vi "PASSCMNdll.vi"(8 "error in (no error)":errorcluster, 11 "Inputs":T2) -> (0 "error out":errorcluster, 3 "Outputs":T1)   [LabVIEW 2016]
doc: "subroutine PASSCMN(hvr, iset, icomp, jcomp, hstr, ilng, dbl, arr, ierr, herr, hvr_length, hstr_length,\nherr_length)\n\nGet or set values of variables in the common blocks.\n\nExamples:\nCall PASSCMN ('txeos', 0,3,0, h,i, tmx,z, ierr,herr) - get tmax of component 3\nCall PASSCMN ('deos', 1,2,0, h,i, dmx,z, ierr,herr) - set dmax of component 2\nCall PASSCMN ('tz', 0,1,0, h,i, tc, z, ierr,herr) - get reducing temperature of component 1\nCall PASSCMN ('ntermf', 0,1,0, h,nt,v, z, ierr,herr) - get number of terms in the Helmholtz equation for component 1\nCall PASSCMN ('coefhmx',1,1,0, h,i, v, cf, ierr,herr) - set the coefficients in the Helmholtz equation for component 1\nCall PASSCMN ('cpc0', 1,5,0, h,i, v, cp0, ierr,herr) - set the coefficients in the cp0 equation for component 5\nCall PASSCMN ('fprkij', 1,1,2, h,i, v, fpr, ierr,herr) - set the PR coefficient for the 1,2 binary\n\nINPUTS:\nhvr --character string with the common variable's name (lower case only)\niset --flag to indicate the get/set condition\n 0 - get variable value\n 1 - set variable value\nicomp --component number\njcomp --second component number for binary mixture variables\nhstr --input for a character string\nilng --input for a long variable\ndbl --input for a double precision variable\narr --input for a double precision array\n note: values in this array are not initialized to 0\n\nOUTPUTS:\nhstr -- output for a character string\nilng -- output for a long variable\ndbl -- output for a double precision variable\narr -- output for a double precision array\n note: values in this array are not initialized to 0\nierr -- error flag: \n 0 = successful\n 1 = unrecognized variable name\nherr -- error string (character*255 variable if ierr<>0)\nhvr_length -- length of variable hvr (default: -1)\nhstr_length -- length of variable hstr (default: 255)\nherr_length -- length of variable herr (default: 255)"
uses:
  REFPROP.DLL
panel:
  # "REFPROP-PASSCMNdll.vi"
  # "void  PASSCMN(CStr hvr, int32_t *iset, int32_t *icomp, int32_t *jcomp, CStr hstr, int32_t *iling, double *dbl, double *arr, int32_t *ierr, CStr herr, int32_t hvr_length, int32_t hstr_length, int32_t herr_length)"
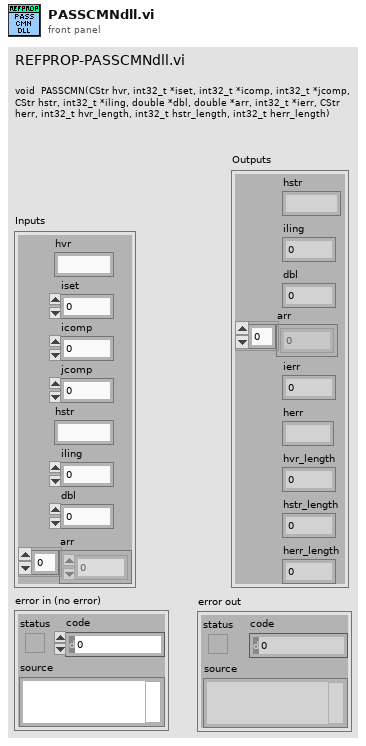
[diagram p1: front panel]
types:
  T1 = cluster{"hstr":string, "iling":i32, "dbl":dbl, "arr":dbl[], "ierr":i32, "herr":string, "hvr_length":i32, "hstr_length":i32, "herr_length":i32}
  T2 = cluster{"hvr":string, "iset":i32, "icomp":i32, "jcomp":i32, "hstr":string, "iling":i32, "dbl":dbl, "arr":dbl[]}
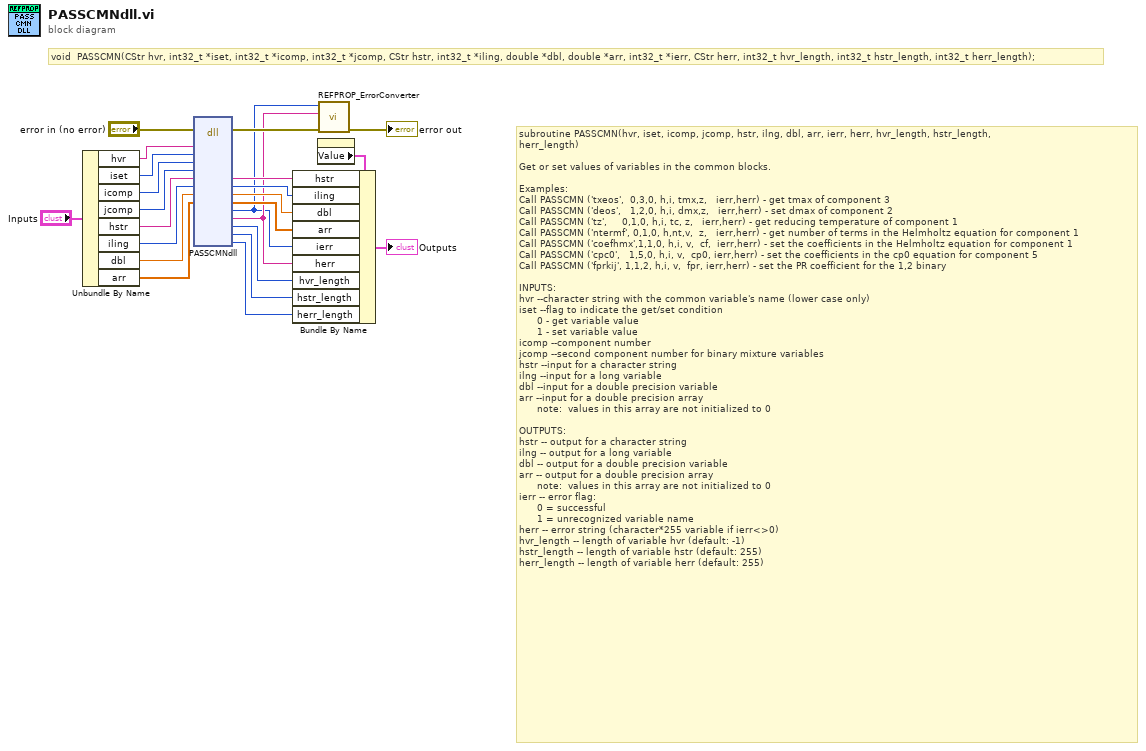
[diagram p0: block diagram]
diagram:
  # "void  PASSCMN(CStr hvr, int32_t *iset, int32_t *icomp, int32_t *jcomp, CStr hstr, int32_t *iling, double *dbl, double *arr, int32_t *ierr, CStr herr, int32_t hvr_length, int32_t hstr_length, int32_t herr_length);"
  # "subroutine PASSCMN(hvr, iset, icomp, jcomp, hstr, ilng, dbl, arr, ierr, herr, hvr_length, hstr_length,\nherr_length)\n\nGet or set values of variables in the common blocks.\n\nExamples:\nCall PASSCMN ('txeos',  0,3,0, h,i, tmx,z,   ierr,herr) - get tmax of component 3\nCall PASSCMN ('deos',   1,2,0, h,i, dmx,z,   ierr,herr) - set dmax of component 2\nCall PASSCMN ('tz',     0,1,0, h,i, tc, z,   ierr,herr) - get reducing temperature of component 1\nCall PASSCMN ('ntermf', 0,1,0, h,nt,v,  z,   ierr,herr) - get number of terms in the Helmholtz equation for component 1\nCall PASSCMN ('coefhmx',1,1,0, h,i, v,  cf,  ierr,herr) - set the coefficients in the Helmholtz equation for component 1\nCall PASSCMN ('cpc0',   1,5,0, h,i, v,  cp0, ierr,herr) - set the coefficients in the cp0 equation for component 5\nCall PASSCMN ('fprkij', 1,1,2, h,i, v,  fpr, ierr,herr) - set the PR coefficient for the 1,2 binary\n\nINPUTS:\nhvr --character string with the common variable's name (lower case only)\niset --flag to indicate the get/set condition\n      0 - get variable value\n      1 - set variable value\nicomp --component number\njcomp --second component number for binary mixture variables\nhstr --input for a character string\nilng --input for a long variable\ndbl --input for a double precision variable\narr --input for a double precision array\n      note:  values in this array are not initialized to 0\n\nOUTPUTS:\nhstr -- output for a character string\nilng -- output for a long variable\ndbl -- output for a double precision variable\narr -- output for a double precision array\n      note:  values in this array are not initialized to 0\nierr -- error flag: \n      0 = successful\n      1 = unrecognized variable name\nherr -- error string (character*255 variable if ierr<>0)\nhvr_length -- length of variable hvr (default: -1)\nhstr_length -- length of variable hstr (default: 255)\nherr_length -- length of variable herr (default: 255)"
  n1 = Unbundle By Name("Inputs") -> ("hvr"=w19:string, "iset"=w18:i32, "icomp"=w17:i32, "jcomp"=w16:i32, "hstr"=w15:string, "iling"=w14:i32, "dbl"=w13:dbl, "arr"=w12:dbl[])
  n2 = dll-call lib="S:/009 - Testing/02 - Performance Testing/REFPROP/REFPROP.*" fn="PASSCMNdll"(error in="error in (no error)", "hvr"=w19, "iset"=w18, "icomp"=w17, "jcomp"=w16, "hstr"=w15, "iling"=w14, "dbl"=w13, "arr"=w12) -> (error out=w23:errorcluster, "hstr"=w4:string, "iling"=w5:i32, "dbl"=w6:dbl, "arr"=w7:dbl[], "ierr"=w1:i32, "herr"=w2:string, "hvr_length"=w8:i32, "hstr_length"=w9:i32, "herr_length"=w10:i32)  [unwired: 12 in, 1 out]
  n3 = property on="Outputs" class="Clust (strict)"() -> ("Value"=w11:T1)  [unwired: 2 in, 2 out]
  n4 = Bundle By Name(cluster=w11, "hstr"=w4, "iling"=w5, "dbl"=w6, "arr"=w7, "ierr"=w1, "herr"=w2, "hvr_length"=w8, "hstr_length"=w9, "herr_length"=w10) -> (→"Outputs":T1)
  n5 = call "REFPROP_ErrorConverter.vi"("error in (no error)"=w23, "Error Message"=w2, "Error Code"=w1) -> ("error out"=→"error out":errorcluster)  [unwired: 8 in]
